vi "Add User Attribute.vi"(0 "User Configuration Manager in":refnum<class "User Configuration Manager.lvclass">, 5 "Username":string, 7 "Attribute Name":string, 9 "Attribute Value":variant, 11 "error in (no error)":errorcluster) -> (4 "User Configuration Manager out":refnum<class "User Configuration Manager.lvclass">, 8 "Replaced":bool, 15 "error out":errorcluster)   [LabVIEW 2017, in "User Configuration Manager.lvlib" / "User Configuration Manager.lvclass"]
doc: "Adds an attribute to the user."
uses:
  User Configuration Manager.lvclass
  User Configuration Manager.lvclass/User Configuration Manager.ctl
  6731e4c8-f3e8-4323-a82b-686f1038a7fb.vi
  Accessors/Read Linked List Ref .vi
  <vilib>/gpm_packages/@cs/linked-list/Source/Linked List/ILinkedList/ILinked List.lvclass
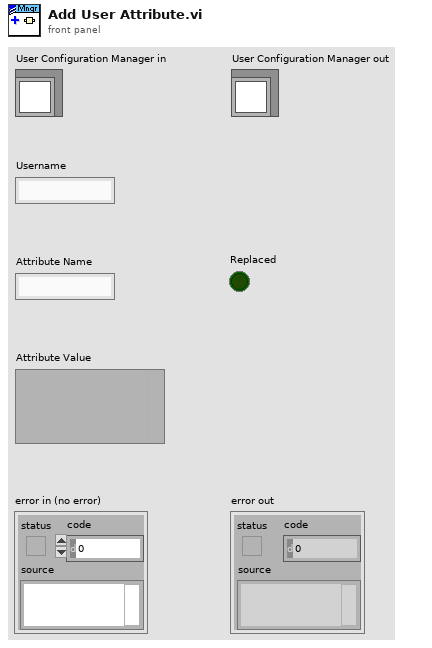
[diagram p1: front panel]
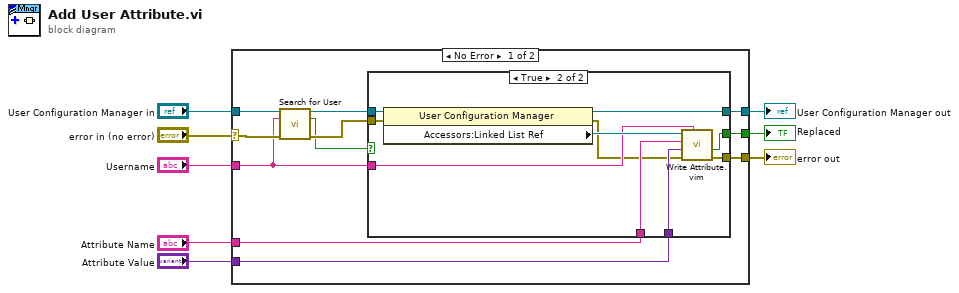
[diagram p0: block diagram]
diagram:
  n1 = case shown="No Error" "error in (no error)" {
    selector: "error in (no error)" -> [w10 w32]
    tunnel: "User Configuration Manager in" -> [w14 w33]
    tunnel: "Attribute Name" -> [w18 _]
    tunnel: "Username" -> [w9 _]
    tunnel: [w19 w33] -> w5
    tunnel: [w15 w32] -> w4
    tunnel: "Attribute Value" -> [w17 _]
    tunnel: [w16 _] -> w1
    frame No Error {
      n2 = call-dynamic "Search for User.vi"("User Configuration Manager in"=w14, "Username"=w9, "error in (no error)"=w10) -> ("User Configuration Manager out"=w13:refnum<class "User Configuration Manager.lvclass">, "Found"=w11:bool, "error out"=w12:errorcluster)  [unwired: 10 in]
      n3 = case shown="True" w11 {
        tunnel: w13 -> [w21 w31]
        tunnel: [w21 w30] -> w19
        tunnel: w12 -> [w20 w29]
        tunnel: w9 -> [_ w27]
        tunnel: w18 -> [_ w26]
        tunnel: w17 -> [_ w25]
        tunnel: [_ w23] -> w16
        tunnel: [w20 w22] -> w15
        frame False {
        }
        frame True {
          n4 = property class="User Configuration Manager"(reference=w31, error in=w29) -> (reference out=w30:refnum<class "User Configuration Manager.lvclass">, error out=w24:errorcluster, "Accessors:Linked List Ref "=w28:refnum<data-value>)
          n5 = call "Write Attribute.vim"("Linked List ID"=w27, "error in (no error)"=w24, "Attribute"=w25, "Attribute Name"=w26, "Linked List Ref"=w28) -> ("error out"=w22:errorcluster, "Replaced?"=w23:bool)  [unwired: 3 in, 2 out]
        }
      }
    }
    frame Error {
    }
  }
  "error out" <- w4
  "User Configuration Manager out" <- w5
  "Replaced" <- w1
